vi "MT Detect PAM.vi"(5 "input complex waveform":T3={"t0"=0.0, "dt"=1.0, "Y"=[]} {"Y" format="%.3f"; "dt" format="%^.2e"; "t0" format="%.4f"}, 7 "PAM system parameters":T2={"samples per symbol (16)"=16, "symbol map"=[]} {"symbol map" format="%.3f"}, 9 "synchronization parameters":T1 {"sync sequence" format="%.2f"}, 11 "error in (no error)":errorcluster, 12 "matched filter coefficients":dbl[](array[numeric]) format="%.2f", 13 "reset? (T)":bool=TRUE, 14 "flush buffers? (F)":bool) -> (6 "output bit stream":i8[](array[numeric]), 10 "sync found index (symbols)":dbl format="%.4f", 15 "error out":errorcluster)   [LabVIEW 2020, in "niDMT.lvlib"]
doc: "Demodulates a pulse-amplitude-modulated (PAM) complex baseband waveform and returns the demodulated bit stream. This VI attempts to remove carrier and phase offset by locking to the carrier signal."
uses:
  <vilib>/addons/Modulation/niDMT.lvlib
  <vilib>/addons/Modulation/Analog/controls/Complex Data Waveform.ctl
  <vilib>/Utility/error.llb/Error Cluster From Error Code.vi
  <vilib>/addons/Modulation/Digital/Support/Common/mod_Truncate FIR Filter (complex).vi
  <vilib>/addons/Modulation/niAMT.lvlib
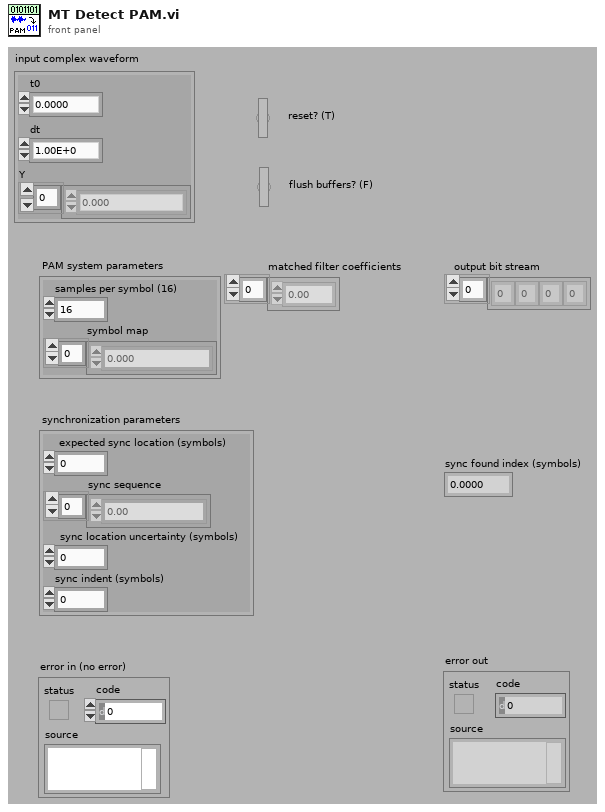
[diagram p1: front panel]
types:
  T1 = cluster{"expected sync location (symbols)":i32, "sync sequence":cdb[], "sync location uncertainty (symbols)":i32, "sync indent (symbols)":i32}
  T2 = cluster{"samples per symbol (16)":i32, "symbol map":cdb[]}
  T3 = typedef "niAMT.lvlib/Complex Data Waveform.ctl" = cluster{"t0":dbl, "dt":dbl, "Y":cdb[]}
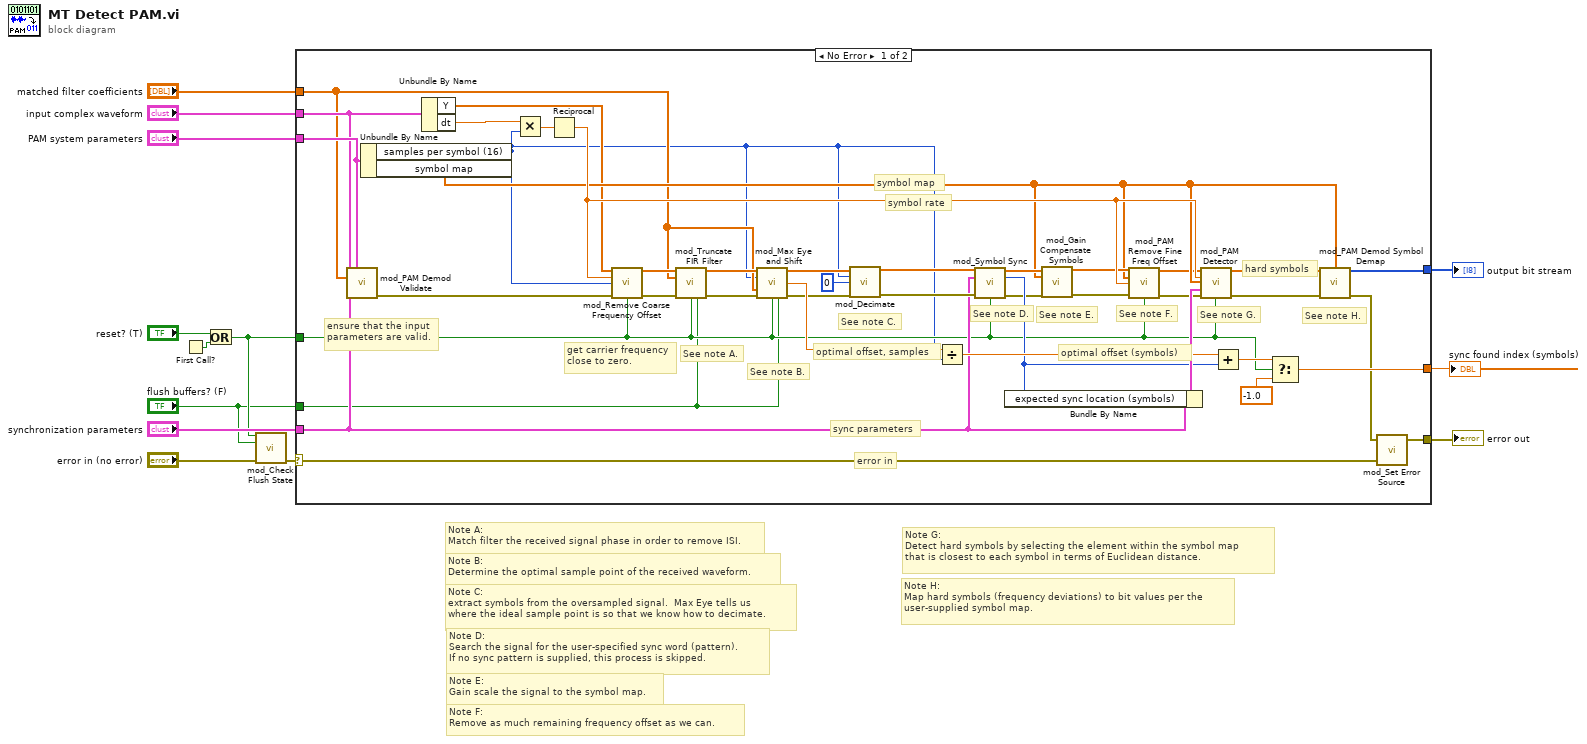
[diagram p0: block diagram]
diagram:
  # "Note E:\nGain scale the signal to the symbol map."
  # "Note H:\nMap hard symbols (frequency deviations) to bit values per the \nuser-supplied symbol map."
  # "Note D:\nSearch the signal for the user-specified sync word (pattern).  \nIf no sync pattern is supplied, this process is skipped."
  # "Note F:\nRemove as much remaining frequency offset as we can."
  # "Note C:\nextract symbols from the oversampled signal.  Max Eye tells us \nwhere the ideal sample point is so that we know how to decimate."
  # "Note B:\nDetermine the optimal sample point of the received waveform."
  # "Note A:\nMatch filter the received signal phase in order to remove ISI."
  # "Note G:\nDetect hard symbols by selecting the element within the symbol map \nthat is closest to each symbol in terms of Euclidean distance."
  n1 = First Call?() -> (First Call?: T/F=w6:bool)
  n2 = Or(x="reset? (T)", y=w6) -> (x .or. y?=w3:bool)
  n3 = call <vilib>:"mod_Check Flush State.vi"("reset?"=w3, "flush buffers? (F)"="flush buffers? (F)", "error in (no error)"="error in (no error)") -> ("error out"=w4:errorcluster)  [unwired: 12 out]
  n4 = case shown="No Error" w4 {
    selector: w4 -> [w29 w55]
    tunnel: w3 -> [w32 _]
    tunnel: "input complex waveform" -> [w37 _]
    tunnel: [w28 w55] -> w7
    tunnel: "matched filter coefficients" -> [w17 _]
    tunnel: [w54 _] -> w9
    tunnel: [w38 _] -> w8
    tunnel: "PAM system parameters" -> [w51 _]
    tunnel: "synchronization parameters" -> [w43 _]
    tunnel: "flush buffers? (F)" -> [w14 _]
    frame No Error {
      # "See note H."
      # "symbol rate"
      # "hard symbols"
      # "sync parameters"
      # "error in"
      # "symbol map"
      # "See note E."
      # "See note G."
      # "See note D."
      # "See note F."
      # "See note C."
      # "get carrier frequency close to zero."
      # "ensure that the input parameters are valid."
      # "See note B."
      # "See note A."
      # "optimal offset (symbols)"
      # "optimal offset, samples"
      n5 = call <vilib>:"mod_PAM Demod Validate.vi"("Input Complex Waveform"=w37, "PAM System Parameters"=w51, "Matched Filter Coefficients"=w17, "Synchronization Parameters"=w43) -> ("error out"=w45:errorcluster)  [unwired: 11 out]
      n6 = Unbundle By Name(w51) -> ("samples per symbol (16)"=w15:i32, "symbol map"=w23:cdb[])
      n7 = Unbundle By Name(w37) -> ("Y"=w16:cdb[], "dt"=w48:dbl)
      n8 = Multiply(x=w48, y=w15) -> (x*y=w49:dbl)
      n9 = Reciprocal(x=w49) -> (1/x=w44:dbl)
      n10 = call <vilib>:"mod_Remove Coarse Frequency Offset.vi"("Signal In"=w16, "Symbol Rate, Hz"=w44, "Samples Per Symbol (16)"=w15, "error in (no error)"=w45, "Reset? (T)"=w32) -> ("Signal Out"=w35:cdb[], "error out"=w53:errorcluster)  [unwired: 9 out]
      n11 = call-poly <vilib>:"mod_Truncate FIR Filter.vi"("Signal In"=w35, "Filter Coefficients"=w17, "error in (no error)"=w53, "Reset? (T)"=w32, "flush buffers? (F)"=w14) -> ("Signal Out"=w34:cdb[], "error out"=w46:errorcluster)  [unwired: 7 in, 2 out]
      n12 = call <vilib>:"mod_Max Eye and Shift.vi"("Signal In"=w34, "Samples Per Symbol (16)"=w15, "matched filter coefficients"=w17, "error in (no error)"=w46, "Reset? (T)"=w32, "flush buffers? (F)"=w14) -> ("Signal Out"=w18:cdb[], "Optimal Offset (in Samples)"=w36:dbl, "error out"=w19:errorcluster)  [unwired: 1 in, 6 out]
      n13 = call <vilib>:"mod_Decimate.vi"("Signal In"=w18, "Samples Per Symbol (16)"=w15, "Offset"=0, "error in (no error)"=w19) -> ("Signal Out"=w31:cdb[], "error out"=w50:errorcluster)  [unwired: 1 in, 9 out]
      n14 = Divide(x=w36, y=w15) -> (x/y=w47:dbl)
      n15 = call <vilib>:"mod_Symbol Sync.vi"("Signal In"=w31, "Synchronization Parameters"=w43, "error in (no error)"=w50, "Reset? (T)"=w32) -> ("Signal Out"=w25:cdb[], "Sync Location (symbols)"=w42:i32, "error out"=w27:errorcluster)  [unwired: 1 in, 8 out]
      n16 = Bundle By Name(cluster=w43, "expected sync location (symbols)"=w42) -> (w52:T1)
      n17 = call <vilib>:"mod_Gain Compensate Symbols.vi"("Symbols In"=w25, "Symbol Map"=w23, "error in (no error)"=w27) -> ("Symbols Out"=w24:cdb[], "error out"=w26:errorcluster)  [unwired: 11 out]
      n18 = call <vilib>:"mod_PAM Remove Fine Freq Offset.vi"("Symbols"=w24, "Symbol Map"=w23, "Symbol Rate, Hz"=w44, "error in (no error)"=w26, "Reset? (T)"=w32) -> ("Symbols"=w22:cdb[], "error out"=w41:errorcluster)  [unwired: 9 out]
      n19 = call <vilib>:"mod_PAM Detector.vi"("Signal In"=w22, "Symbol Rate, Hz"=w44, "Symbol Map"=w23, "Synchronization Parameters"=w52, "error in (no error)"=w41, "Reset? (T)"=w32) -> ("Signal Out"=w21:cdb[], "error out"=w20:errorcluster)  [unwired: 8 out]
      n20 = Add(x=w47, y=w42) -> (x+y=w39:dbl)
      n21 = Select(t=w39, s=w32, f=-1.0) -> (s? t:f=w38:dbl)
      n22 = call <vilib>:"mod_PAM Demod Symbol Demap.vi"("Symbols In"=w21, "Symbol Map"=w23, "error in (no error)"=w20) -> ("Bits Out"=w54:i8[], "error out"=w30:errorcluster)  [unwired: 11 out]
      n23 = call <vilib>:"mod_Set Error Source.vi"("initial error in (no error)"=w29, "final error in (no error)"=w30) -> ("error out"=w28:errorcluster)  [unwired: 3 out]
    }
    frame Error {
    }
  }
  "error out" <- w7
  "sync found index (symbols)" <- w8
  "output bit stream" <- w9
